vi "Week2.vi"() -> ()   [LabVIEW 2021]
uses:
  <vilib>/Analysis/2dsp.llb/Power Spectrum (DBL).vi
  <vilib>/numeric/Random Number (Range) DBL.vi
  <vilib>/Analysis/NI_AALPro.lvlib
panel:
  in  "Noise Amplitude":dbl
  in  "Noise Frequency":dbl
  in  "Sine Amplitude":dbl
  in  "Sine Frequency":dbl
  in  "?":bool
  out "Added signal":dynamicdata(graph)
  out "merged signal":dynamicdata(graph)
  in  "Frequency":dbl
  in  "Delay Time (s)":dbl
  in  "?":bool
  out "Power Spectrum of a signal":dbl[](graph)
  in  "?":bool
  out "˚C":dbl(slide) scale=0.0..100.0
  in  "˚K":dbl(slide) scale=25.0..250.0
  out "index_min 2 row":dbl
  out "index_max 2 row":dbl
  out "Array 4":dbl[][](array[numeric])
  out "index_min 2 col":dbl
  out "index_max 2 col":dbl
  out "Min 2":dbl
  out "Max 2":dbl
  out "Array 3":dbl[](array[numeric])
  out "index_min":dbl
  out "index_max":dbl
  out "Min":dbl
  out "Max":dbl
  out "Numeric 3":dbl
  in  "stop 8":bool
  out "˚C":dbl
  in  "˚F":dbl
  out "Waveform Graph 2":dbl[](graph)
  in  "?":bool
  in  "value to add":dbl
  out "Tank 2":dbl(slide) scale=0.0..10.0
  in  "Numeric 4":dbl
  in  "stop 6":bool
  out "result":dbl
  in  "Boolean 2":bool
  in  "Stop bottom":bool
  in  "Slide":dbl(slide) scale=10.0..30.0
  out "High ˚C":bool
  out "Low ˚C":bool
  out "Waveform Chart 4":cluster{"Slide":dbl, i32, i32}(graph)
  out "Waveform Chart 3":dbl[][](graph)
  in  "stop 5":bool
  out "Waveform Chart 2":dbl[][](graph)
  in  "stop 4":bool
  out "Waveform Graph":dbl[](graph)
  in  "stop 3":bool
  out "Waveform Chart":cluster{dbl, dbl}(graph)
  out "Array 2":dbl[][](array[numeric])
  out "Array":dbl[](array[numeric])
  out "Tank":dbl(slide) scale=0.0..10.0
  in  "stop 2":bool
  out "Boolean":bool
  out "Knob":dbl(knob) scale=0.0..10.0
  out "Numeric 2":dbl
  in  "stop":bool
  out "Numeric":dbl
  # "Array 2"
  # "array"
  # "New array"
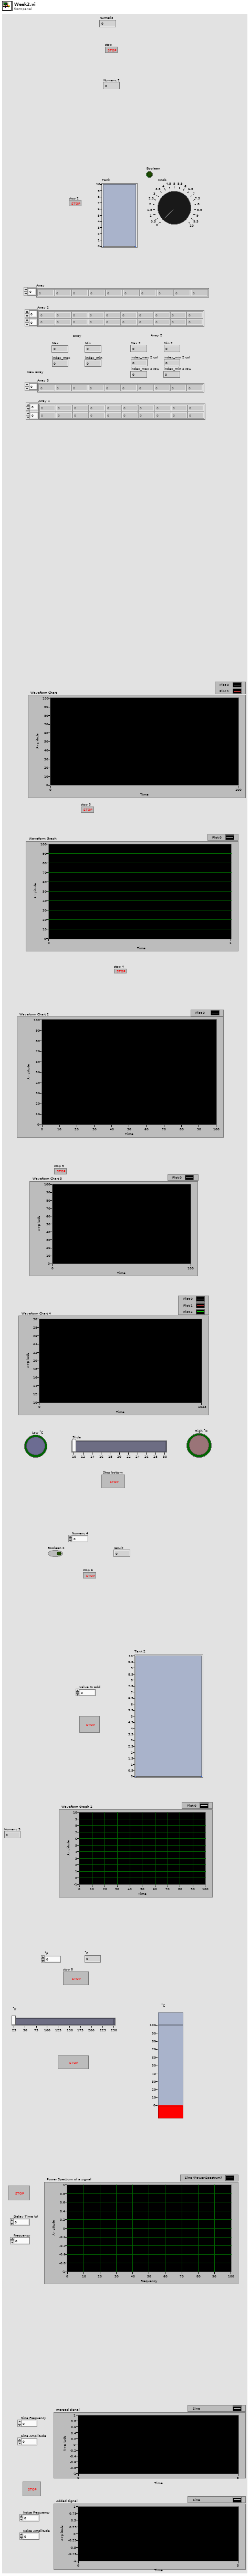
[diagram p1: front panel]
types:
  T1 = typedef "NI_Matrix.lvlib/RealMatrix.ctl" = dbl[][]
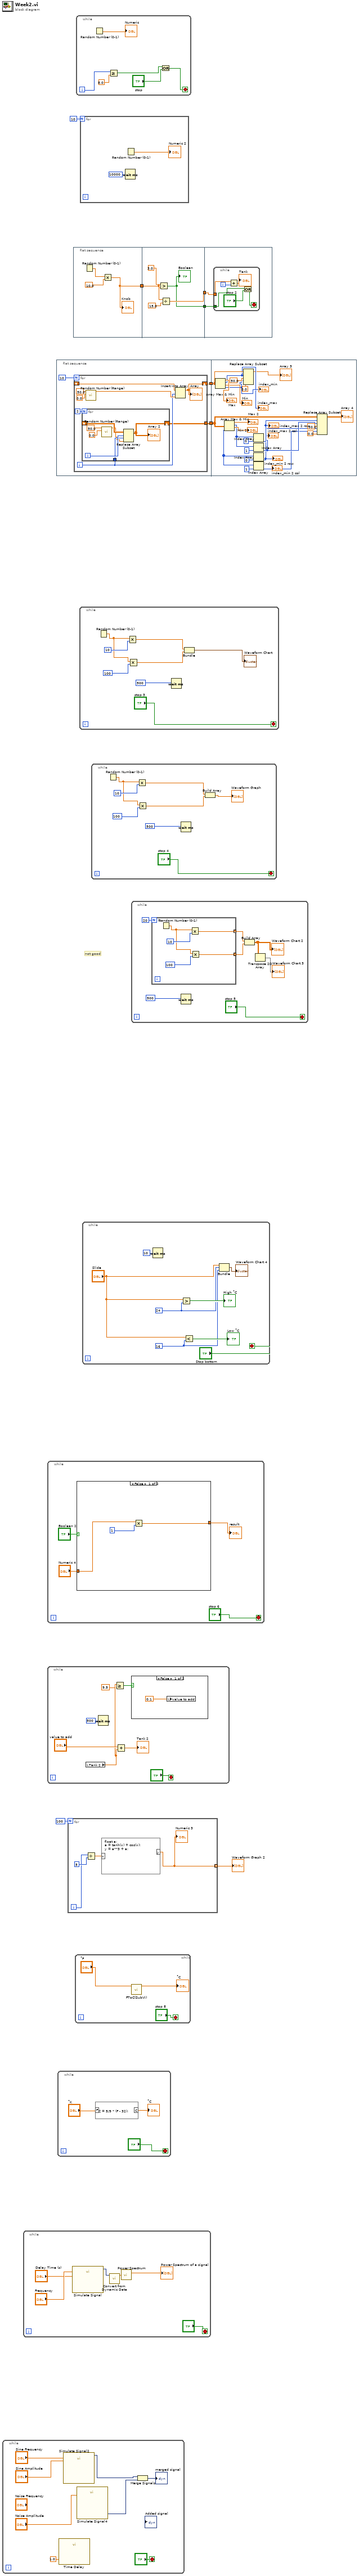
[diagram p0: block diagram]
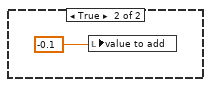
[diagram p2: hidden frame]
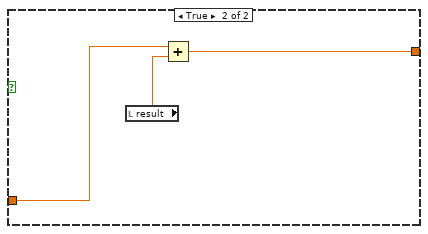
[diagram p3: hidden frame]
diagram:
  # "not good"
  n1 = while {
    stop <- "?" stop-if-true
    n2 = call "Time Delay"("Delay Time (s)"=1.0) -> ()  [unwired: 10 in, 1 out]
    n3 = call "Simulate Signal2"("Frequency"="Sine Frequency", "Amplitude"="Sine Amplitude") -> ("Sine"=w11:dynamicdata)  [unwired: 12 in, 1 out]
    n4 = call "Simulate Signal4"("Noise amplitude"="Noise Amplitude") -> ("DC with Uniform Noise"=w10:dynamicdata)  [unwired: 13 in, 1 out]
    n5 = Merge Signals(w11, w10) -> (→"merged signal":dynamicdata)
  }
  n6 = while {
    stop <- "?" stop-if-true
    n7 = call "Simulate Signal"("Frequency"="Frequency", "Phase"="Delay Time (s)") -> ("Sine"=w19:dynamicdata)  [unwired: 12 in, 1 out]
    n8 = call "Convert from Dynamic Data"("Dynamic Data Type"=w19) -> ("Array"=w18:dbl[])  [unwired: 3 in]
    n9 = call-poly <vilib>:"Power Spectrum.vi"("X"=w18) -> ("Power Spectrum"=→"Power Spectrum of a signal":dbl[])  [unwired: 1 out]
  }
  n10 = while {
    stop <- "?" stop-if-true
    n11 = local read "Tank 2"() -> (w24:dbl)
    n12 = Wait (ms)(milliseconds to wait=u32 500) -> ()  [unwired: 1 out]
    n13 = Greater Or Equal?(x=w24, y=9.5) -> (x >= y?=w25:bool)
    n14 = Add(x="value to add", y=w24) -> (x+y=→"Tank 2":dbl)
    n15 = case shown="False" w25 {
      frame False {
        n16 = local write "value to add"(0.1) -> ()
      }
      frame True {
        n17 = local write "value to add"(-0.1) -> ()
      }
    }
  }
  n18 = while {
    stop <- "stop 6" stop-if-true
    n19 = case shown="False" "Boolean 2" {
      tunnel: [w37 w41] -> w34
      tunnel: "Numeric 4" -> [w36 w40]
      frame False {
        n20 = Multiply(x=w36, y=1) -> (x*y=w37:dbl)
      }
      frame True {
        n21 = local read "result"() -> (w39:dbl)
        n22 = Add(x=w40, y=w39) -> (x+y=w41:dbl)
      }
    }
    "result" <- w34
  }
  n23 = flat-sequence {
    tunnel: [w43] -> w2
    tunnel: [w42] -> w1
    tunnel: w2 -> [w83]
    tunnel: w1 -> [w67]
    frame #0 {
      n24 = for {
        N: 10 -> [_]
        shift-right: [w49] -> w43
        shift-left: _ -> [w48]
        tunnel: [w45] -> w42
        i -> [w46]
        n25 = for {
          N: 2 -> [_]
          shift-right: [w57] -> w45
          shift-left: _ -> [w56]
          tunnel: w46 -> [w54]
          i -> [w55]
          n26 = call-poly <vilib>:"Random Number (Range).vi"("lower bound (0)"=0.0, "upper bound (100)"=50.0) -> ("number"=w53:dbl)  [unwired: 9 in]
          n27 = Replace Array Subset(array=w56, new element=w53, index (row)=w55, index (col)=w54) -> (w57:T1)
          "Array 2" <- w57
        }
        n28 = call-poly <vilib>:"Random Number (Range).vi"("lower bound (0)"=0.0, "upper bound (100)"=50.0) -> ("number"=w50:dbl)  [unwired: 9 in]
        n29 = Insert Into Array(array=w48, index=w46, new element=w50) -> (w49:dbl[])
        "Array" <- w49
      }
    }
    frame #1 {
      n30 = Array Max & Min(array=w83) -> (max value=→"Max":dbl, max index (indices)=w77:i32, min value=→"Min":dbl, min index (indices)=w78:i32)
      "index_min" <- w78
      "index_max" <- w77
      n31 = Array Max & Min(array=w67) -> (max value=→"Max 2":dbl, max index (indices)=w73:i32[], min value=→"Min 2":dbl, min index (indices)=w72:i32[])
      n32 = Replace Array Subset(array=w83, new element #1=50.0, index #1=w77, new element #2=0.0, index #2=w78) -> (→"Array 3":dbl[])
      n33 = Index Array(array=w73, index=0) -> (element=w63:i32)
      "index_max 2 row" <- w63
      n34 = Index Array(array=w73, index=1) -> (element=w62:i32)
      "index_max 2 col" <- w62
      n35 = Index Array(array=w72, index=0) -> (element=w61:i32)
      "index_min 2 row" <- w61
      n36 = Index Array(array=w72, index=1) -> (element=w60:i32)
      "index_min 2 col" <- w60
      n37 = Replace Array Subset(array=w67, new element #1=50.0, index (row) #1=w63, index (col) #1=w62, new element #2=0.0, index (row) #2=w61, index (col) #2=w60) -> (→"Array 4":T1)
    }
  }
  n38 = while {
    stop <- "?" stop-if-true
    n39 = formula code="C = 5/9 * (F - 32);"("F"="˚K") -> ("C"=→"˚C":dbl)
  }
  n40 = for {
    N: 100 -> [_]
    tunnel: [w87] -> w3 mode=indexing
    i -> [w88]
    n41 = Divide(x=w88, y=5) -> (x/y=w90:dbl)
    n42 = formula code="float a;\na = tanh(x) + cos(x);\ny = a**3 + a;"("x"=w90) -> ("y"=w87:dbl)
    "Numeric 3" <- w87
  }
  "Waveform Graph 2" <- w3
  n43 = flat-sequence {
    tunnel: [w91] -> w7
    tunnel: w7 -> [w96]
    tunnel: [w95] -> w6
    tunnel: [w94] -> w5
    tunnel: w6 -> [w100]
    tunnel: w5 -> [w99]
    frame #0 {
      n44 = Random Number (0-1)() -> (number: 0 to 1=w93:dbl)
      n45 = Multiply(x=w93, y=10.0) -> (x*y=w91:dbl)
      "Knob" <- w91
    }
    frame #1 {
      n46 = Greater?(x=3.0, y=w96) -> (0:w94:bool)
      "Boolean" <- w94
      n47 = Divide(x=w96, y=15.0) -> (x/y=w95:dbl)
    }
    frame #2 {
      n48 = while {
        tunnel: w100 -> [w105]
        tunnel: w99 -> [w103]
        i -> [w106]
        stop <- w102 stop-if-true
        n49 = Add(x=w105, y=w106) -> (x+y=→"Tank":dbl)
        n50 = Or(x=w103, y="stop 2") -> (x .or. y?=w102:bool)
      }
    }
  }
  n51 = while {
    stop <- "stop 8" stop-if-true
    n52 = call "FToC(SubVI).vi"("˚F"="˚F") -> ("Numeric"=→"˚C":dbl)  [unwired: 10 in]
  }
  n53 = while {
    i -> [w113]
    stop <- w110 stop-if-true
    n54 = Random Number (0-1)() -> (number: 0 to 1=→"Numeric":dbl)
    n55 = Greater Or Equal?(x=w113, y=8.0) -> (x >= y?=w112:bool)
    n56 = Or(x=w112, y="stop") -> (x .or. y?=w110:bool)
  }
  n57 = while {
    stop <- "stop 3" stop-if-true
    n58 = Random Number (0-1)() -> (number: 0 to 1=w122:dbl)
    n59 = Multiply(x=w122, y=10) -> (x*y=w120:dbl)
    n60 = Multiply(x=w122, y=100) -> (x*y=w119:dbl)
    n61 = Wait (ms)(milliseconds to wait=500) -> ()  [unwired: 1 out]
    n62 = Bundle(w120, w119) -> (→"Waveform Chart":cluster{dbl, dbl})  [unwired: 1 in]
  }
  n63 = for {
    N: 10 -> [_]
    n64 = Wait (ms)(milliseconds to wait=u32 10000) -> ()  [unwired: 1 out]
    n65 = Random Number (0-1)() -> (number: 0 to 1=→"Numeric 2":dbl)
  }
  n66 = while {
    stop <- "Stop bottom" stop-if-true
    w128 = 16
    w129 = 24
    n67 = Wait (ms)(milliseconds to wait=u32 10) -> ()  [unwired: 1 out]
    n68 = Greater?(x="Slide", y=w129) -> (0:→"High ˚C":bool)
    n69 = Less?(x="Slide", y=w128) -> (x < y?=→"Low ˚C":bool)
    n70 = Bundle("Slide"="Slide", w129, w128) -> (→"Waveform Chart 4":cluster{"Slide":dbl, i32, i32})  [unwired: 1 in]
  }
  n71 = while {
    stop <- "stop 4" stop-if-true
    n72 = Random Number (0-1)() -> (number: 0 to 1=w140:dbl)
    n73 = Multiply(x=w140, y=10) -> (x*y=w136:dbl)
    n74 = Multiply(x=w140, y=100) -> (x*y=w135:dbl)
    n75 = Wait (ms)(milliseconds to wait=500) -> ()  [unwired: 1 out]
    n76 = Build Array(w136, w135) -> (→"Waveform Graph":dbl[])
  }
  n77 = while {
    stop <- "stop 5" stop-if-true
    n78 = for {
      N: 20 -> [_]
      tunnel: [w150] -> w147 mode=indexing
      tunnel: [w149] -> w146 mode=indexing
      n79 = Random Number (0-1)() -> (number: 0 to 1=w152:dbl)
      n80 = Multiply(x=w152, y=10) -> (x*y=w150:dbl)
      n81 = Multiply(x=w152, y=100) -> (x*y=w149:dbl)
    }
    n82 = Wait (ms)(milliseconds to wait=500) -> ()  [unwired: 1 out]
    n83 = Build Array(w147, w146) -> (w143:dbl[][])
    "Waveform Chart 2" <- w143
    n84 = Transpose 2D Array(2D array=w143) -> (transposed array=→"Waveform Chart 3":dbl[][])
  }
